vi "TestVisionGear.vi"(10 "R/G/B in":cluster{"Lower value":i32, "Upper value":i32}[](array[cluster])=[{"Lower value"=0, "Upper value"=40}, {"Lower value"=80, "Upper value"=255}, {"Lower value"=0, "Upper value"=255}], 11 "Refnum in":T1) -> ()   [LabVIEW 2016]
uses:
  <vilib>/vision/Image Controls.llb/IMAQ Image.ctl
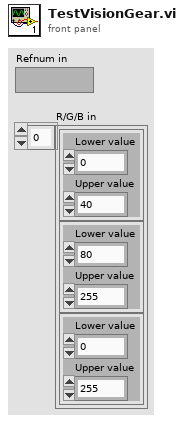
[diagram p1: front panel]
types:
  T1 = typedef "IMAQ Image.ctl" = refnum<image>
  T2 = cluster{"Left":dbl, "Top":dbl, "Right":dbl, "Bottom":dbl}
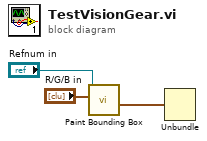
[diagram p0: block diagram]
diagram:
  n1 = call "Paint Bounding Box.vi"("Camera Image"="Refnum in", "R/G/B"="R/G/B in") -> ("Bounding Box Final"=w1:T2)  [unwired: 5 in, 4 out]
  n2 = Unbundle(w1) -> ()  [unwired: 4 out]
